vi "LV to ITX  Retrieve (TDMS).vi"(4 "Action":enum16{"Read Wavenames", "Read Data"}(ring), 8 "error in (no error)":errorcluster, 9 "Channels":cluster{"X":string, "Y":string, "N":string}, 10 "File or Folder Path":path=path "C:/", 11 "LVtoITX.lvclass":refnum<class "LVtoITX.lvclass">) -> (0 "error out":errorcluster, 1 "Parameter(s)":dbl[](array[numeric]), 2 "X vs Y":cluster{dbl[], dbl[]}[](graph), 3 "LVtoITX.lvclass out":refnum<class "LVtoITX.lvclass">)   [LabVIEW 2016, in "LVtoITX.lvclass"]
uses:
  LVtoITX.lvclass
  <userlib>/LevyLab/Graph Utilities/graph_utilities.lvclass/graph_utilities.ctl
  <userlib>/LevyLab/Graph Utilities/graph_utilities.lvclass
panel:
  in  "Channels 2":cluster{"X":u16, "Y":u16, "N":u16} {"N" items=["time", "temp", "B", "AI1", "AI2", "AI3", "AI4", "AI5", "AI6", "AO1", "AO2", "AO3", "AO4"]; "Y" items=["time", "temp", "B", "AI1", "AI2", "AI3", "AI4", "AI5", "AI6", "AO1", "AO2", "AO3", "AO4"]; "X" items=["time", "temp", "B", "AI1", "AI2", "AI3", "AI4", "AI5", "AI6", "AO1", "AO2", "AO3", "AO4"]}
  in  "y name":string="A y name"
  in  "x name":string="B x name"
  in  "recolor traces?":bool
  out "Comments":string
  out "Path":path
  in  "length":i32=1
  out "counter":i32
  in  "offset":i32
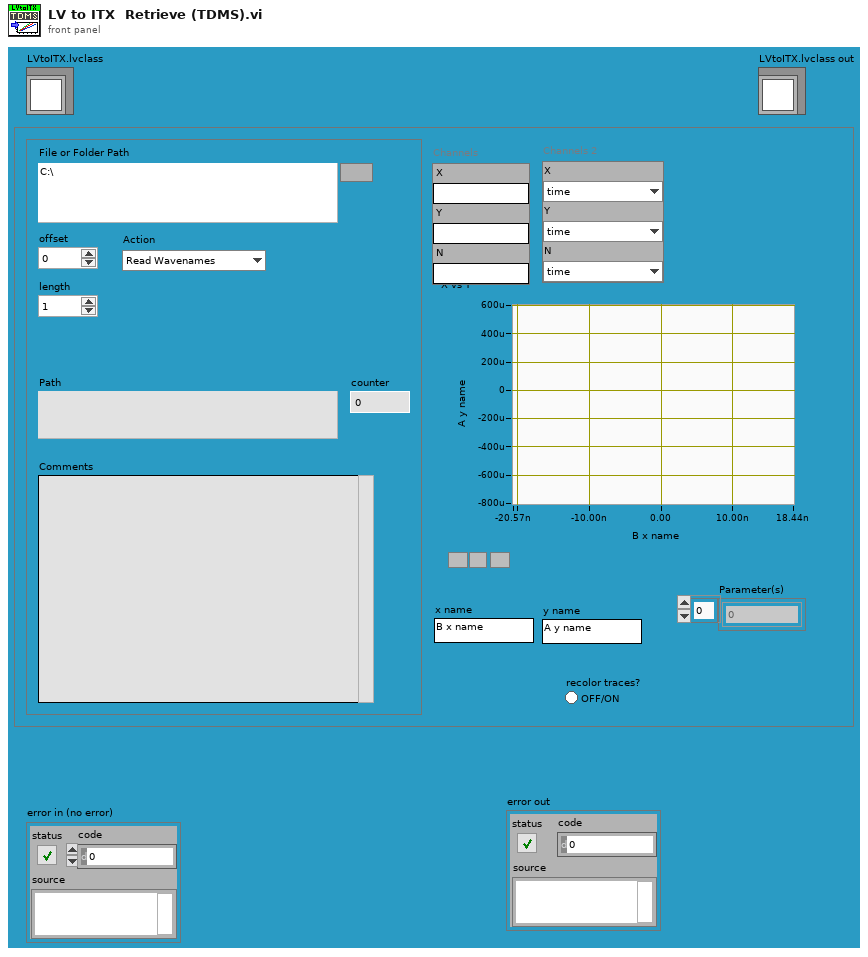
[diagram p1: front panel]
types:
  T1 = enum32{"Bad", "Idle", "Run top level", "Running"}
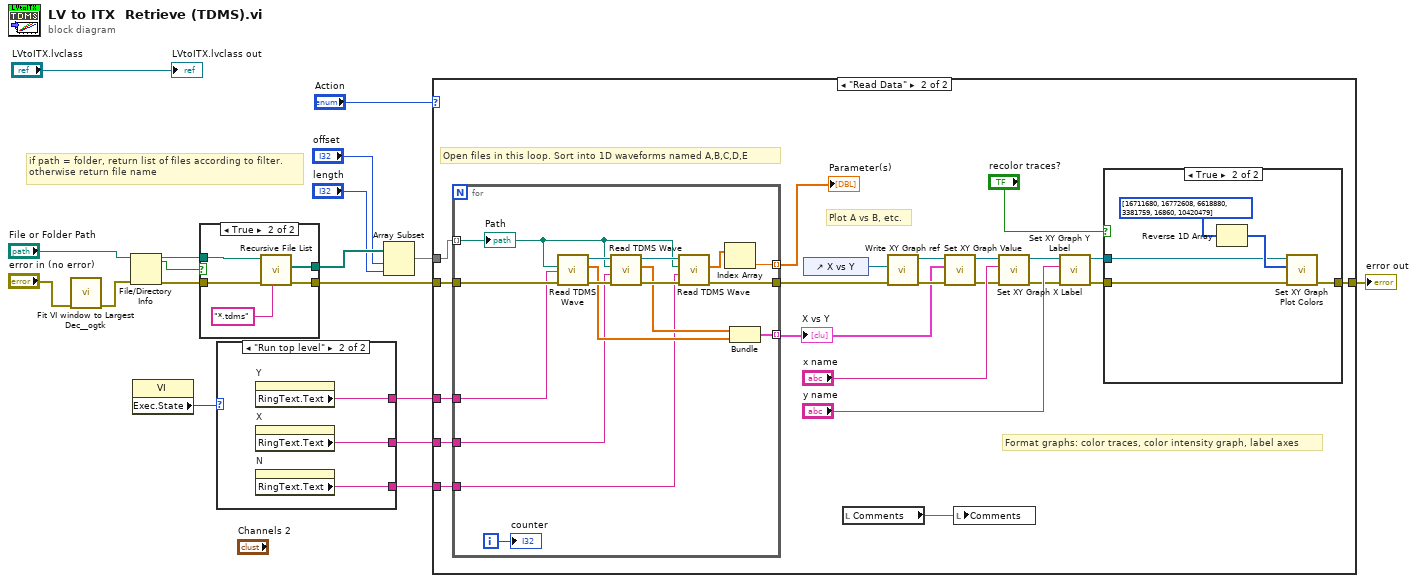
[diagram p0: block diagram]
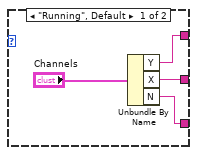
[diagram p2: hidden frame]
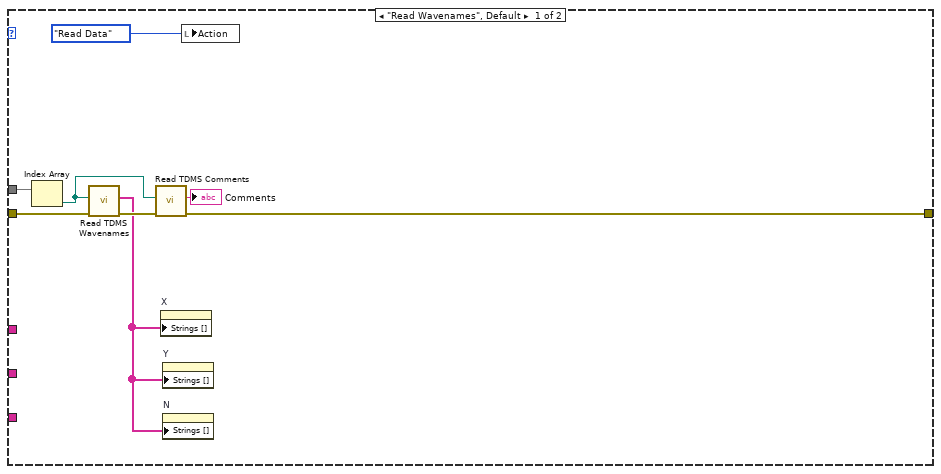
[diagram p3: hidden frame]
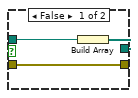
[diagram p5: hidden frame]
diagram:
  # "if path = folder, return list of files according to filter.\notherwise return file name"
  n1 = call <userlib>:"Fit VI window to Largest Dec__ogtk.vi"("error in (no error)"="error in (no error)") -> ("error out"=w5:errorcluster)  [unwired: 5 in, 1 out]
  n2 = File/Directory Info(path="File or Folder Path", error in=w5) -> (path out=w10:path, directory=w12:bool, error out=w11:errorcluster)  [unwired: 4 out]
  n3 = property class="VI"() -> ("Exec.State"=w4:T1)  [unwired: 2 in, 2 out]
  n4 = case shown="True" w12 {
    tunnel: [w21 w25] -> w18
    tunnel: w10 -> [w20 w26]
    tunnel: w11 -> [w19 w24]
    tunnel: [w19 w23] -> w13
    frame False {
      n5 = Build Array(w20) -> (w21:path[])
    }
    frame True {
      n6 = call <vilib>:"Recursive File List.vi"("pattern"="*.tdms", "error in (no error)"=w24, "Folder Path"=w26) -> ("error out"=w23:errorcluster, "All Files in Dir"=w25:path[])  [unwired: 4 in, 3 out]
    }
  }
  n7 = case shown="\"Run top level\"" w4 {
    tunnel: [w27 w33] -> w3
    tunnel: [w29 w32] -> w2
    tunnel: [w28 w31] -> w1
    frame "Running", Default {
      n8 = Unbundle By Name("Channels") -> ("Y"=w27:string, "X"=w29:string, "N"=w28:string)
    }
    frame "Run top level" {
      n9 = property on="Y" class="Ring (strict)"() -> ("RingText.Text"=w33:string)  [unwired: 2 in, 2 out]
      n10 = property on="X" class="Ring (strict)"() -> ("RingText.Text"=w32:string)  [unwired: 2 in, 2 out]
      n11 = property on="N" class="Ring (strict)"() -> ("RingText.Text"=w31:string)  [unwired: 2 in, 2 out]
    }
  }
  n12 = Array Subset(array=w18, index="offset", length="length") -> (w15:path[])
  n13 = case shown="\"Read Data\"" "Action" {
    tunnel: w15 -> [w41 w48]
    tunnel: w13 -> [w40 w63]
    tunnel: [w36 w47] -> w6
    tunnel: w3 -> [_ w44]
    tunnel: w2 -> [_ w43]
    tunnel: w1 -> [_ w42]
    frame "Read Wavenames", Default {
      n14 = Index Array(array=w41) -> (element=w35:path)  [unwired: 1 in]
      n15 = call "Read TDMS Wavenames.vi"("error in (no error)"=w40, "path"=w35) -> ("error out"=w39:errorcluster, "Wavenames"=w34:string[])  [unwired: 7 in, 1 out]
      n16 = call "Read TDMS Comments.vi"("error in (no error)"=w39, "path"=w35) -> ("error out"=w36:errorcluster, "Comments"=→"Comments":string)  [unwired: 7 in, 1 out]
      n17 = property on="X" class="Ring (strict)"("Strings []"=w34) -> ()  [unwired: 2 in, 2 out]
      n18 = property on="Y" class="Ring (strict)"("Strings []"=w34) -> ()  [unwired: 2 in, 2 out]
      n19 = property on="N" class="Ring (strict)"("Strings []"=w34) -> ()  [unwired: 2 in, 2 out]
      n20 = local write "Action"(enum16{"Read Wavenames", "Read Data"}."Read Data" ("Enum")) -> ()
    }
    frame "Read Data" {
      # "Plot A vs B, etc."
      # "Format graphs: color traces, color intensity graph, label axes"
      # "Open files in this loop. Sort into 1D waveforms named A,B,C,D,E"
      n21 = for {
        tunnel: w48 -> [w70] mode=indexing
        tunnel: [w78] -> w59 mode=indexing
        tunnel: w63 -> [w77]
        tunnel: [w71] -> w45 mode=indexing
        tunnel: [w69] -> w46
        tunnel: w44 -> [w66]
        tunnel: w43 -> [w65]
        tunnel: w42 -> [w64]
        i -> [w79]
        n22 = call "Read TDMS Wave.vi"("error in (no error)"=w77, "channel name(s) in"=w66, "path"=w70) -> ("error out"=w76:errorcluster, "data"=w67:dbl[], "LVtoITX out"=w75:refnum<class "LVtoITX.lvclass">)  [unwired: 6 in]
        n23 = call "Read TDMS Wave.vi"("error in (no error)"=w76, "channel name(s) in"=w65, "path"=w70, "LVtoITX in"=w75) -> ("error out"=w74:errorcluster, "data"=w68:dbl[], "LVtoITX out"=w73:refnum<class "LVtoITX.lvclass">)  [unwired: 5 in]
        n24 = call "Read TDMS Wave.vi"("error in (no error)"=w74, "channel name(s) in"=w64, "path"=w70, "LVtoITX in"=w73) -> ("error out"=w69:errorcluster, "data"=w72:dbl[])  [unwired: 5 in, 1 out]
        n25 = Index Array(array=w72) -> (element=w71:dbl)  [unwired: 1 in]
        n26 = Bundle("data"=w68, "data"=w67) -> (w78:cluster{"data":dbl[], "data":dbl[]})  [unwired: 1 in]
        "counter" <- w79
        "Path" <- w70
      }
      "X vs Y" <- w59
      "Parameter(s)" <- w45
      n27 = control-ref of="X vs Y"() -> (w61:refnum<vi>)
      n28 = local read "Comments"() -> (w49:string)
      n29 = call <userlib>:"Write XY Graph ref.vi"("error in (no error)"=w46, "XY Graph"=w61) -> ("error out"=w60:errorcluster, "graph_utilities out"=w56:refnum<class "graph_utilities.lvclass">)  [unwired: 8 in]
      n30 = call <userlib>:"Set XY Graph Value.vi"("error in (no error)"=w60, "Value"=w59, "graph_utilities in"=w56) -> ("error out"=w54:errorcluster, "graph_utilities out"=w55:refnum<class "graph_utilities.lvclass">)  [unwired: 7 in]
      n31 = local write "Comments"(w49) -> ()
      n32 = call <userlib>:"Set XY Graph X Label.vi"("error in (no error)"=w54, "X Label"="x name", "graph_utilities in"=w55) -> ("error out"=w52:errorcluster, "graph_utilities out"=w53:refnum<class "graph_utilities.lvclass">)  [unwired: 7 in]
      n33 = call <userlib>:"Set XY Graph Y Label.vi"("error in (no error)"=w52, "Y Label"="y name", "graph_utilities in"=w53) -> ("error out"=w50:errorcluster, "graph_utilities out"=w51:refnum<class "graph_utilities.lvclass">)  [unwired: 7 in]
      n34 = case shown="True" "recolor traces?" {
        tunnel: w51 -> [_ w84]
        tunnel: w50 -> [w80 w83]
        tunnel: [w80 w81] -> w47
        frame False {
        }
        frame True {
          n35 = Reverse 1D Array(array=u32[] [16711680, 16772608, 6618880, 3381759, 16860, 10420479] ("color scale")) -> (reversed array=w85:u32[])
          n36 = call <userlib>:"Set XY Graph Plot Colors.vi"("error in (no error)"=w83, "Colors []"=w85, "graph_utilities in"=w84) -> ("error out"=w81:errorcluster)  [unwired: 7 in, 1 out]
        }
      }
    }
  }
  "error out" <- w6
  "LVtoITX.lvclass out" <- "LVtoITX.lvclass"
